vi "Prepare_Initial_Output_States.vi"() -> ()   [LabVIEW 2021]
uses:
  Pulse_Sequence_Global.vi
panel:
  in  "End configuration":bool
  in  "Initial states":T1(array[cluster])
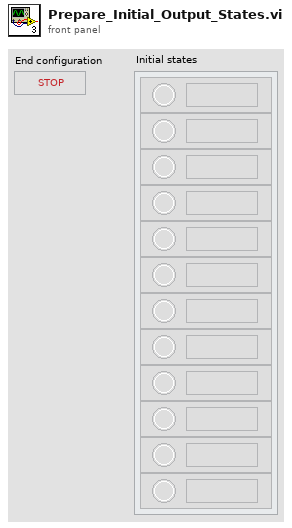
[diagram p1: front panel]
types:
  T1 = cluster{"Type of channel":string, "Boolean":bool}[]
  T2 = typedef "Channel_Cluster.ctl" = cluster{"Channel name":string, "Channel":u8}
  T3 = cluster{"Type of channel":string, "Boolean":bool}
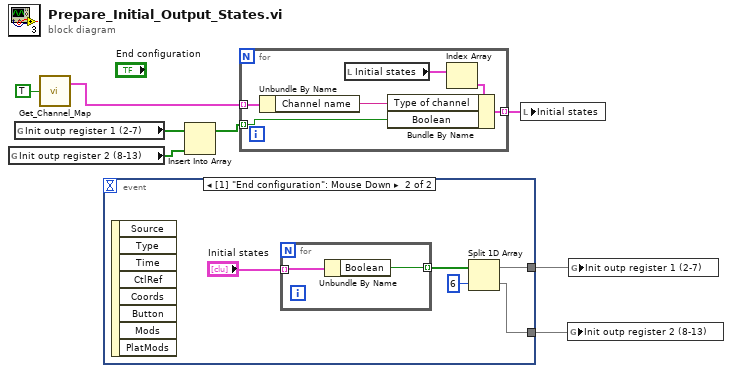
[diagram p0: block diagram]
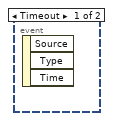
[diagram p2: hidden frame]
diagram:
  n1 = global read "Pulse_Sequence_Global.vi" "Init outp register 2 (8-13)"() -> (w4:bool[])
  n2 = global read "Pulse_Sequence_Global.vi" "Init outp register 1 (2-7)"() -> (w5:bool[])
  n3 = call "Get_Channel_Map.vi"("Get default(?)"=TRUE) -> ("Channels map"=w2:T2[])  [unwired: 2 in, 1 out]
  n4 = event shown="[1] \"End configuration\": Mouse Down" {
    selector: _ -> [_ _]
    dyn-events: _ -> [_ _]
    timeout: _ -> [_ _]
    tunnel: [_ w10] -> w7
    tunnel: [_ w9] -> w6
    event Timeout {
      n5 = event-data() -> ()  [unwired: 1 in, 3 out]
    }
    event "End configuration": Mouse Down {
      n6 = event-data() -> ()  [unwired: 1 in, 8 out]
      n7 = for {
        tunnel: "Initial states" -> [w15] mode=indexing
        tunnel: [w14] -> w13 mode=indexing
        n8 = Unbundle By Name(w15) -> ("Boolean"=w14:bool)
      }
      n9 = Split 1D Array(array=w13, index=6) -> (first subarray=w10:bool[], second subarray=w9:bool[])
    }
  }
  n10 = Insert Into Array(array=w5, new element=w4) -> (w3:bool[])  [unwired: 1 in]
  n11 = for {
    tunnel: w2 -> [w19] mode=indexing
    tunnel: [w17] -> w8 mode=indexing
    tunnel: w3 -> [w16] mode=indexing
    n12 = Unbundle By Name(w19) -> ("Channel name"=w18:string)
    n13 = local read "Initial states"() -> (w21:T1)
    n14 = Index Array(array=w21) -> (element=w20:T3)  [unwired: 1 in]
    n15 = Bundle By Name(cluster=w20, "Type of channel"=w18, "Boolean"=w16) -> (w17:T3)
  }
  n16 = local write "Initial states"(w8) -> ()
  n17 = global write "Pulse_Sequence_Global.vi" "Init outp register 2 (8-13)"(w6) -> ()
  n18 = global write "Pulse_Sequence_Global.vi" "Init outp register 1 (2-7)"(w7) -> ()
